vi "Datadashboard CD GUID Lookup.vi"() -> ()   [LabVIEW 2013, in "Datadashboard CD Custom Device.lvlib"]
doc: "Use this Global VI to access the GUIDs assigned to the page resources of the Custom Device."
uses:
  Datadashboard CD Custom Device.lvlib
panel:
  in  "Custom Device":string="3f6e11e3-fcb1-45cc-b022-d269b60be372"
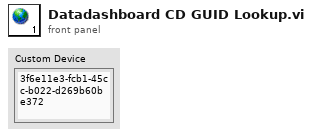
[diagram p1: front panel]
diagram:
